vi "Get Application Version Number.vi"(10 "Number to Strip":i32, 11 "Initial Path":path) -> (0 "error out":errorcluster, 3 "Version":string)   [LabVIEW 2016]
doc: "Retrieve the LV version number of the given application."
panel:
  in  "error in":errorcluster
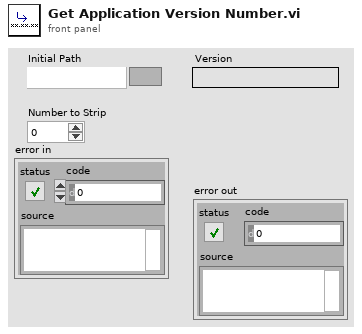
[diagram p1: front panel]
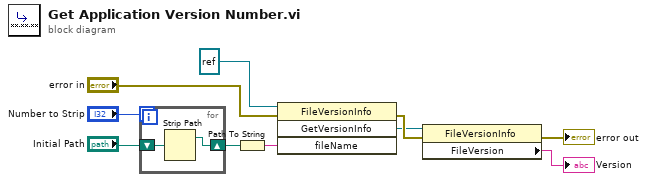
[diagram p0: block diagram]
diagram:
  n1 = for {
    N: "Number to Strip" -> [_]
    shift-right: [w11] -> w9
    shift-left: "Initial Path" -> [w12]
    n2 = Strip Path(path=w12) -> (stripped path=w11:path)  [unwired: 1 out]
  }
  n3 = Path To String(path=w9) -> (string=w5:string)
  n4 = invoke class="FileVersionInfo" method="GetVersionInfo"(reference=refnum<k24> refnum, error in="error in", "fileName"=w5) -> (error out=w6:errorcluster, "GetVersionInfo"=w3:refnum<k24>)  [unwired: 1 in, 2 out]
  n5 = property class="FileVersionInfo"(reference=w3, error in=w6) -> (error out=→"error out":errorcluster, "FileVersion"=→"Version":string)  [unwired: 1 out]
